vi "From PCM task.vi"(10 "PCM input task":T1) -> (2 "task":u64)   [LabVIEW 2022 SP3, in "DAAG task conversion.lvlib"]
uses:
  DAAG task conversion.lvlib
  <vilib>/PDM Acquisition Toolkit/host/Classes/Tasks/PCM Input/PCM Input Task.lvclass
  <vilib>/PDM Acquisition Toolkit/host/Classes/Tasks/PCM Input/Controls/DVR PCM Input Task.ctl
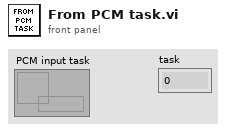
[diagram p1: front panel]
types:
  T1 = typedef "PDM Acquisition Class Library.lvlib/PCM Input Task.lvclass/DVR PCM Input Task.ctl" = refnum<data-value>
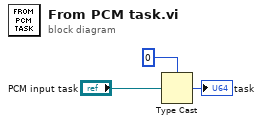
[diagram p0: block diagram]
diagram:
  n1 = Type Cast(type=u64 0, x="PCM input task") -> (*(type *) &x=→"task":u64)
